vi "test_advanced_Doppler_filtered_M_stripped.vi"() -> ()   [LabVIEW 2009]
doc: "Copyright (C) 2009, Stepan A. Baranov\nweb: http://www.OCTLab.org/\nemail: stepan@baranov.su"
uses:
  OCTLib.dll
panel:
  out "version":string
  out "name":string
  out "error out":errorcluster
  out "max":dbl
  out "min":dbl
  out "offset":i32
  out "strip size":i32
  out "width":i32
  out "height":i32
  in  "Small/Big":bool
  out "loop #":i32
  out "RSM_STAT time":u32
  out "LabView time":u32
  out "RSM_STAT Array":dbl[][](array[numeric])
  out "LabView Array":dbl[][](array[numeric])
  in  "stop":bool
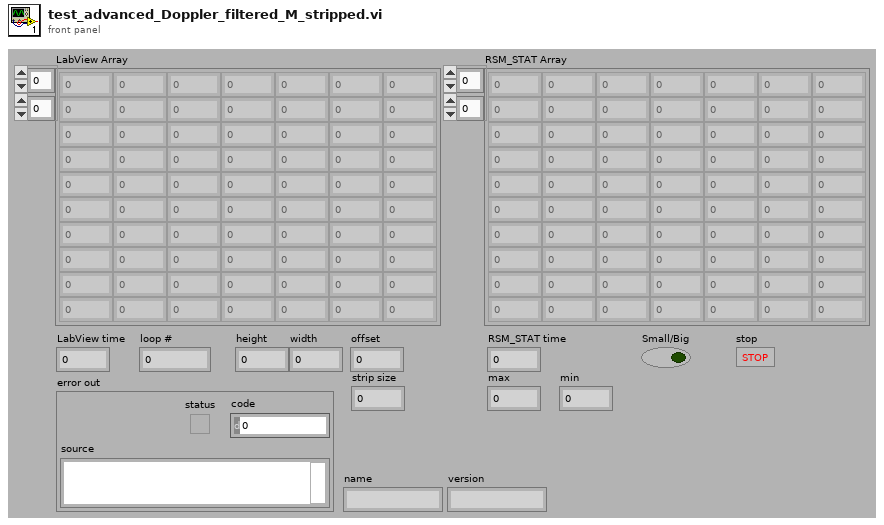
[diagram p1: front panel]
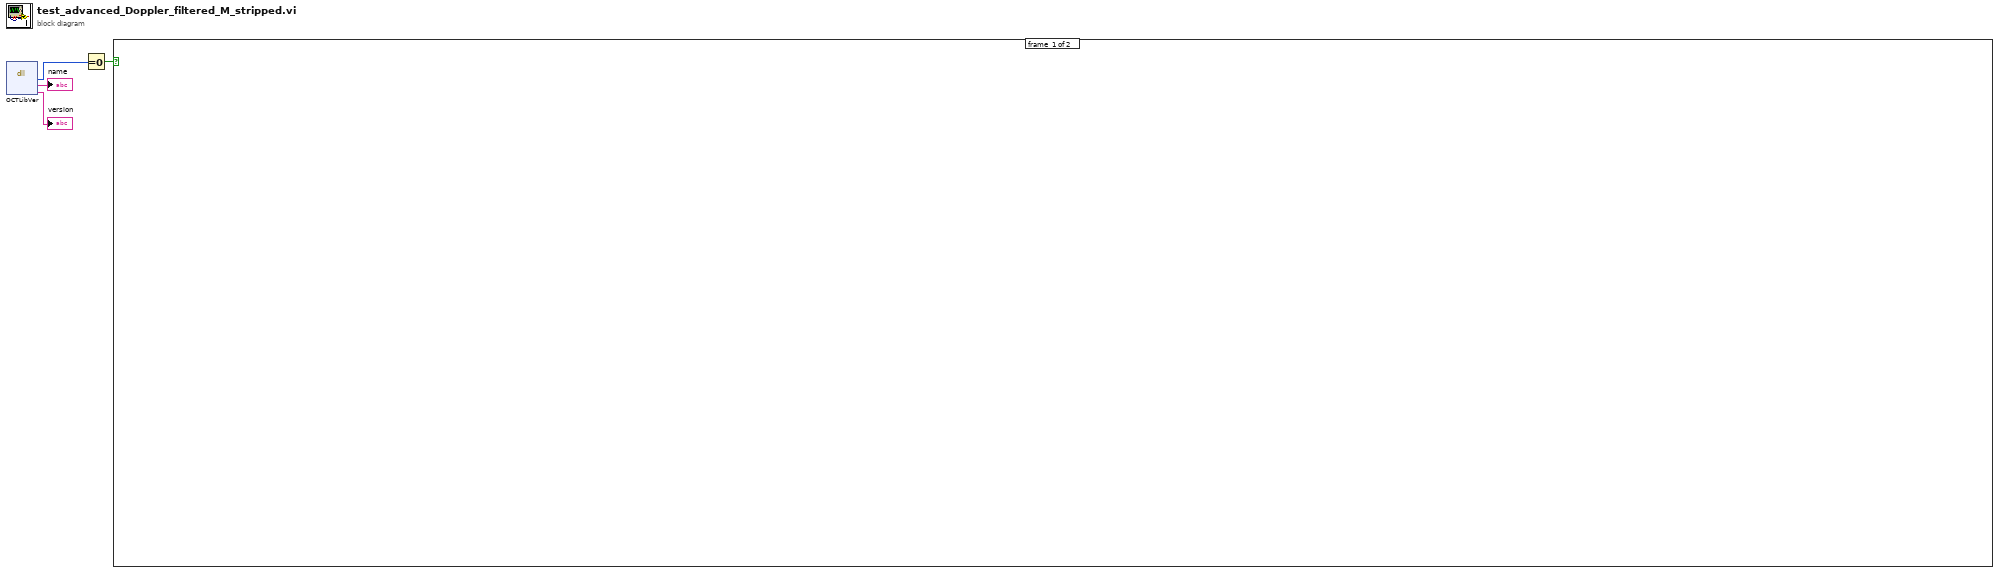
[diagram p0: block diagram]
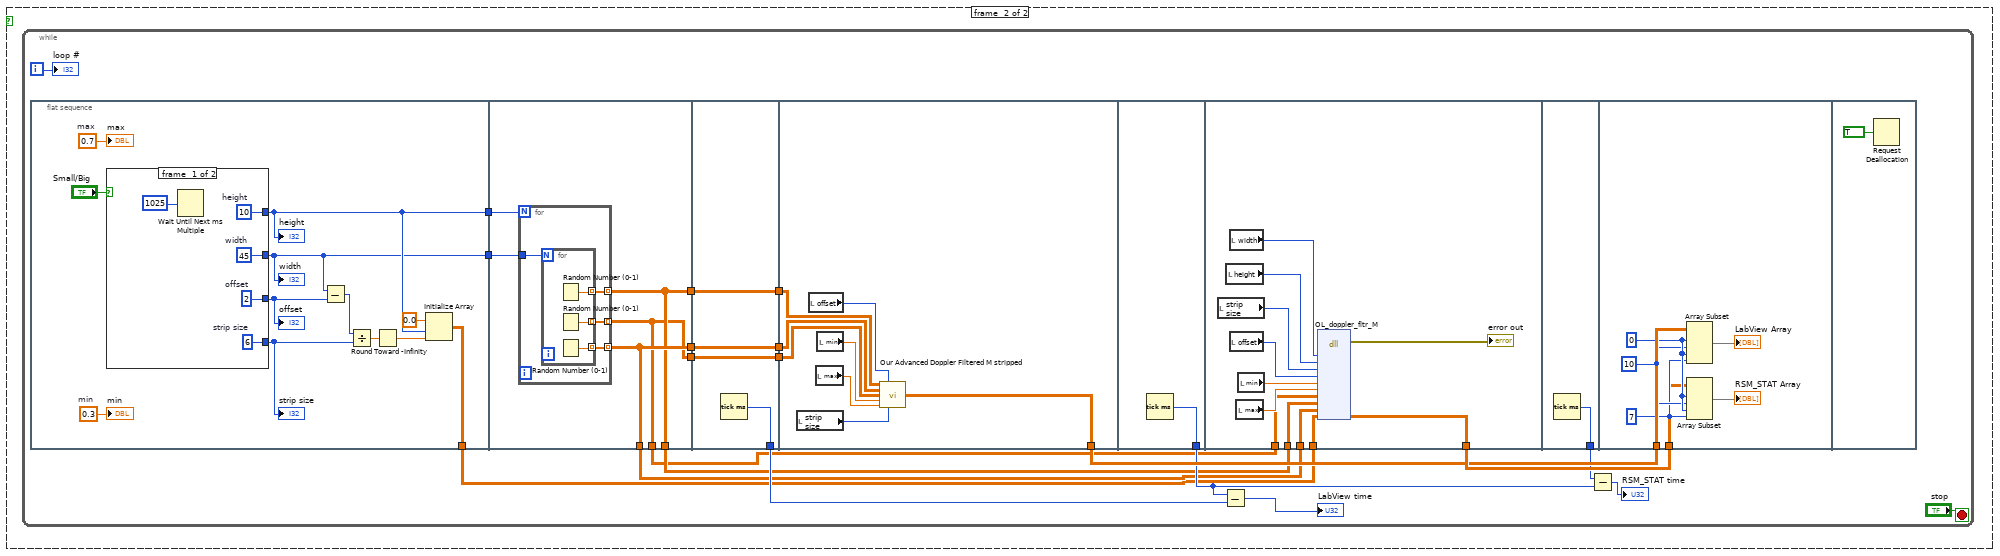
[diagram p2: hidden frame]
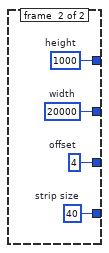
[diagram p3: hidden frame]
diagram:
  n1 = dll-call lib="OCTLib.dll" fn="OCTLibVer"() -> ("status"=w4:i8, "name"=→"name":string, "version"=→"version":string)  [unwired: 5 in, 2 out]
  n2 = Equal To 0?(x=w4) -> (x = 0?=w1:bool)
  n3 = case shown="True" w1 {
    frame #0 {
    }
    frame #1 {
      n4 = while {
        i -> [w17]
        stop <- "stop" stop-if-true
        n5 = flat-sequence {
          tunnel: [w29] -> w13
          tunnel: [w32] -> w12
          tunnel: [w35] -> w8
          tunnel: [w49] -> w16
          tunnel: [w49] -> w14
          tunnel: w13 -> [w51]
          tunnel: w12 -> [w50]
          tunnel: [w48] -> w11
          tunnel: [w48] -> w9
          tunnel: [w47] -> w7
          tunnel: [w47] -> w5
          tunnel: [w62] -> w22
          tunnel: [w61] -> w15
          tunnel: w14 -> [w61]
          tunnel: w11 -> [w59]
          tunnel: [w59] -> w10
          tunnel: w7 -> [w60]
          tunnel: [w60] -> w6
          tunnel: [w70] -> w23
          tunnel: w15 -> [w65]
          tunnel: w10 -> [w67]
          tunnel: w6 -> [w66]
          tunnel: [w71] -> w19
          tunnel: w16 -> [w80]
          tunnel: [w83] -> w24
          tunnel: w9 -> [w79]
          tunnel: w8 -> [w78]
          tunnel: w5 -> [w75]
          tunnel: [w84] -> w20
          tunnel: w24 -> [w85]
          tunnel: w23 -> [w91]
          frame #0 {
            w33 = 0.7  # max
            w34 = 0.3  # min
            n6 = case shown="True" "Small/Big" {
              tunnel: [w41 w46] -> w32
              tunnel: [w42 w45] -> w29
              tunnel: [w39 w44] -> w27
              tunnel: [w38 w43] -> w28
              frame #0 {
                w38 = 2  # offset
                w39 = 6  # strip size
                w42 = 45  # width
                w41 = 10  # height
                n7 = Wait Until Next ms Multiple(millisecond multiple=u32 1025) -> ()  [unwired: 1 out]
              }
              frame #1 {
                w43 = 4  # offset
                w44 = 40  # strip size
                w45 = 20000  # width
                w46 = 1000  # height
              }
            }
            "height" <- w32
            "width" <- w29
            "strip size" <- w27
            "offset" <- w28
            n8 = Subtract(x=w29, y=w28) -> (x-y=w31:i32)
            n9 = Divide(x=w31, y=w27) -> (x/y=w30:dbl)
            n10 = Round Toward -Infinity(1:w30) -> (0:w26:dbl)
            n11 = Initialize Array(0.0 ("element"), w32, w26) -> (w35:dbl[][])
            "min" <- w34
            "max" <- w33
          }
          frame #1 {
            n12 = for {
              N: w50 -> [_]
              tunnel: w51 -> [w55]
              tunnel: [w54] -> w49 mode=indexing
              tunnel: [w53] -> w48 mode=indexing
              tunnel: [w52] -> w47 mode=indexing
              n13 = for {
                N: w55 -> [_]
                tunnel: [w58] -> w54 mode=indexing
                tunnel: [w57] -> w53 mode=indexing
                tunnel: [w56] -> w52 mode=indexing
                n14 = Random Number (0-1)() -> (number: 0 to 1=w57:dbl)
                n15 = Random Number (0-1)() -> (number: 0 to 1=w56:dbl)
                n16 = Random Number (0-1)() -> (number: 0 to 1=w58:dbl)
              }
            }
          }
          frame #2 {
            n17 = Tick Count (ms)() -> (millisecond timer value=w62:u32)
          }
          frame #3 {
            n18 = local read "strip size"() -> (w63:i32)
            n19 = local read "offset"() -> (w64:i32)
            n20 = local read "max"() -> (w68:dbl)
            n21 = local read "min"() -> (w69:dbl)
            n22 = call "Our Advanced Doppler Filtered M stripped.vi"("Real Part"=w67, "Offset"=w64, "Imaginary Part"=w65, "intensity"=w66, "min"=w69, "max"=w68, "Strip Size"=w63) -> ("2D Doppler Image"=w70:dbl[][])  [unwired: 8 in]
          }
          frame #4 {
            n23 = Tick Count (ms)() -> (millisecond timer value=w71:u32)
          }
          frame #5 {
            n24 = local read "strip size"() -> (w73:i32)
            n25 = local read "height"() -> (w81:i32)
            n26 = local read "width"() -> (w82:i32)
            n27 = local read "offset"() -> (w72:i32)
            n28 = local read "max"() -> (w77:dbl)
            n29 = local read "min"() -> (w76:dbl)
            n30 = dll-call lib="OCTLib.dll" fn="OL_doppler_fltr_M"("width"=w82, "height"=w81, "strip size"=w73, "offset"=w72, "min"=w76, "max"=w77, "intensity"=w75, "Re"=w79, "Im"=w80, "data"=w78) -> (error out=→"error out":errorcluster, "data"=w83:dbl[][])  [unwired: 13 in, 1 out]
          }
          frame #6 {
            n31 = Tick Count (ms)() -> (millisecond timer value=w84:u32)
          }
          frame #7 {
            w88 = 10 ("length")
            w87 = 7 ("length")
            w89 = 0 ("index")
            n32 = Array Subset(array=w91, index (row)=w89, length (row)=w88, index (col)=w89, length (col)=w87) -> (→"LabView Array":dbl[][])
            n33 = Array Subset(array=w85, index (row)=w89, length (row)=w88, index (col)=w89, length (col)=w87) -> (→"RSM_STAT Array":dbl[][])
          }
          frame #8 {
            n34 = Request Deallocation(TRUE ("flag")) -> ()
          }
        }
        n35 = Subtract(x=w19, y=w22) -> (x-y=→"LabView time":u32)
        n36 = Subtract(x=w20, y=w19) -> (x-y=→"RSM_STAT time":u32)
        "loop #" <- w17
      }
    }
  }
